vi "Bank - Race Condition.vi"() -> ()   [LabVIEW 2014]
doc: "This VI simulates the transactions that occur in a bank and demonstrates race conditions.\n\nRun the VI, and attempt a simultaneous transaction and notice that either the withdrawal or deposit is lost. Try to find and solve the problem."
panel:
  out "Balance":dbl
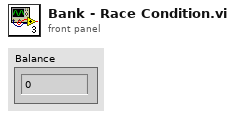
[diagram p1: front panel]
types:
  T1 = typedef "Account Info.ctl" = cluster{"Bank Rendezvous":T2, "Withdrawal Queue":refnum<queue>, "Deposit Queue":refnum<queue>}
  T2 = typedef "Rendezvous RefNum" = refnum<k1>
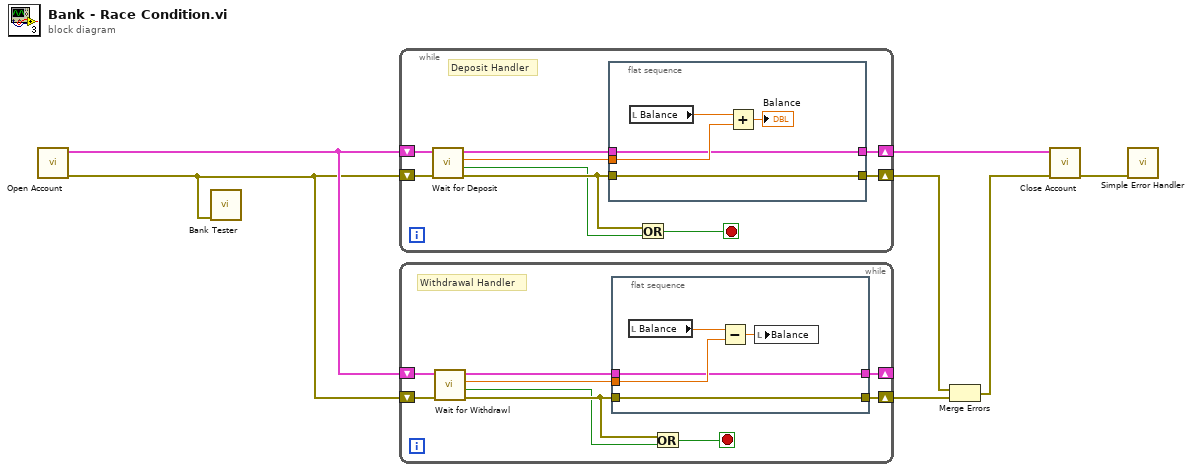
[diagram p0: block diagram]
diagram:
  n1 = call "Open Account.vi"() -> ("error out"=w1:errorcluster, "Account info"=w7:T1)  [unwired: 10 in]
  n2 = call "Bank Tester.vi"("error in"=w1) -> ()  [unwired: 10 in, 1 out]
  n3 = while {
    shift-right: [w12] -> w4
    shift-left: w7 -> [w15]
    shift-right: [w11] -> w6
    shift-left: w1 -> [w14]
    stop <- w8 stop-if-true
    # "Deposit Handler"
    n4 = call "Wait for Deposit.vi"("error in"=w14, "Account info"=w15) -> ("error out"=w10:errorcluster, "Stop?"=w9:bool, "Deposit Amount"=w16:dbl, "Account info out"=w13:T1)  [unwired: 6 in]
    n5 = flat-sequence {
      tunnel: w16 -> [w21]
      tunnel: [w18] -> w12
      tunnel: w13 -> [w18]
      tunnel: w10 -> [w17]
      tunnel: [w17] -> w11
      frame #0 {
        n6 = local read "Balance"() -> (w19:dbl)
        n7 = Add(x=w19, y=w21) -> (x+y=→"Balance":dbl)
      }
    }
    n8 = Or(x=w10, y=w9) -> (x .or. y?=w8:bool)
  }
  n9 = while {
    shift-right: [w26] -> _
    shift-left: w7 -> [w29]
    shift-right: [w25] -> w5
    shift-left: w1 -> [w28]
    stop <- w22 stop-if-true
    # "Withdrawal Handler"
    n10 = call "Wait for Withdrawl.vi"("error in"=w28, "Account info"=w29) -> ("error out"=w24:errorcluster, "Stop?"=w23:bool, "Withdrawal Amount"=w30:dbl, "Account info out"=w27:T1)  [unwired: 6 in]
    n11 = flat-sequence {
      tunnel: w30 -> [w33]
      tunnel: w27 -> [w32]
      tunnel: w24 -> [w31]
      tunnel: [w32] -> w26
      tunnel: [w31] -> w25
      frame #0 {
        n12 = local read "Balance"() -> (w34:dbl)
        n13 = Subtract(x=w34, y=w33) -> (x-y=w35:dbl)
        n14 = local write "Balance"(w35) -> ()
      }
    }
    n15 = Or(x=w24, y=w23) -> (x .or. y?=w22:bool)
  }
  n16 = Merge Errors(w6, w5) -> (w2:errorcluster)
  n17 = call "Close Account.vi"("error in"=w2, "Account info"=w4) -> ("error out"=w3:errorcluster)  [unwired: 9 in]
  n18 = call <vilib>:"Simple Error Handler.vi"("error in (no error)"=w3) -> ()  [unwired: 4 in, 5 out]
